vi "Write Encoder.vi"(10 "Encoder":i32, 11 "ValveModbus in":refnum<class "NeedleValve.lvclass">) -> (3 "ValveModbus out":refnum<class "NeedleValve.lvclass">)   [LabVIEW 2019, in "NeedleValve.lvclass"]
uses:
  NeedleValve.lvclass
  NeedleValve.lvclass/NeedleValve.ctl
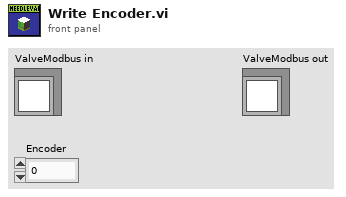
[diagram p1: front panel]
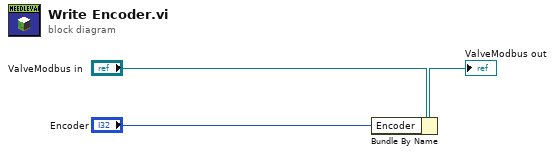
[diagram p0: block diagram]
diagram:
  n1 = Bundle By Name(cluster="ValveModbus in", "Encoder"="Encoder") -> (→"ValveModbus out":refnum<class "NeedleValve.lvclass">)
